vi "Initialize MeasurementLink Session.vi"(7 "remote connection options":T2, 8 "error in":errorcluster, 9 "initialize and close session behavior":T1, 10 "session initialization parameters":T3, 11 "session factory in":refnum<class "Session Factory.lvclass">) -> (0 "error out":errorcluster, 2 "session out":variant, 3 "session factory out":refnum<class "Session Factory.lvclass">)   [LabVIEW 2020, in "IVI Scope Instrument.lvlib" / "Session Factory.lvclass"]
doc: "Creates a new session using the provided <b>session initialization parameters</b>. If the session represents a remote session, <b>initialize and close session behavior</b> determines whether creating the local session creates a new session on the server or attaches to an existing session on the server."
uses:
  Session Factory.lvclass
  <vilib>/MeasurementLink/MeasurementLink Instrument/ISession Factory/Session Initialization Parameters.ctl
  <vilib>/MeasurementLink/MeasurementLink Instrument/ISession Factory/Remote Connection Options.ctl
  <vilib>/MeasurementLink/MeasurementLink Instrument/ISession Factory/Initialize and Close Session Behavior.ctl
  Session Factory.lvclass/Session Factory.ctl
  <vilib>/MeasurementLink/MeasurementLink Instrument/ISession Factory/ISession Factory.lvclass
  <vilib>/ivi/iviscope/_iviscope.llb/IviScope Initialize With Options.vi
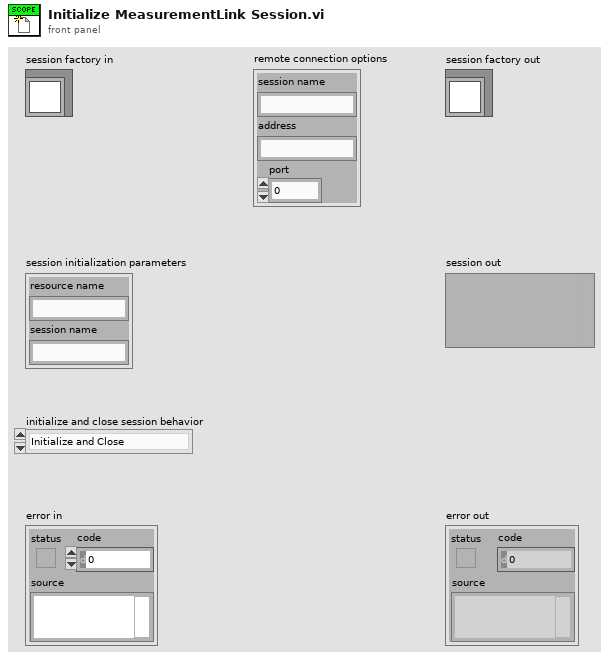
[diagram p1: front panel]
types:
  T1 = typedef "MeasurementLink Instrument.lvlib/ISession Factory.lvclass/Initialize and Close Session Behavior.ctl" = enum16{"Initialize and Close", "Attach and Detach", "Initialize and Detach", "Attach and Close"}
  T2 = typedef "MeasurementLink Instrument.lvlib/ISession Factory.lvclass/Remote Connection Options.ctl" = cluster{"session name":string, "address":string, "port":u32}
  T3 = typedef "MeasurementLink Instrument.lvlib/ISession Factory.lvclass/Session Initialization Parameters.ctl" = cluster{"resource name":string, "session name":string}
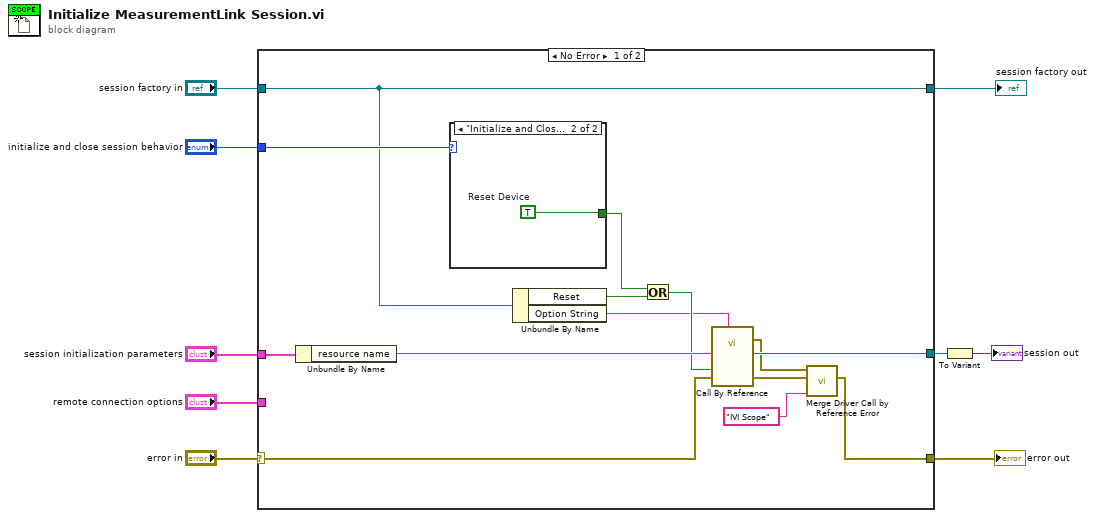
[diagram p0: block diagram]
diagram:
  n1 = case shown="No Error" "error in" {
    selector: "error in" -> [w16 w26]
    tunnel: [w13 w26] -> w8
    tunnel: [w11 w25] -> w7
    tunnel: "session factory in" -> [w11 w25]
    tunnel: "session initialization parameters" -> [w23 _]
    tunnel: [w21 _] -> w3
    tunnel: "initialize and close session behavior" -> [w20 _]
    tunnel: "remote connection options" -> [_ _]
    frame No Error {
      n2 = Unbundle By Name(w23) -> ("resource name"=w22:string)
      n3 = case shown="\"Initialize and Close\", \"Initialize and Detach\"" w20 {
        tunnel: [_ w24] -> w19
        frame Default {
        }
        frame "Initialize and Close", "Initialize and Detach" {
          w24 = TRUE  # Reset Device
        }
      }
      n4 = Unbundle By Name(w11) -> ("Reset"=w18:bool, "Option String"=w10:string)
      n5 = Or(x=w19, y=w18) -> (x .or. y?=w17:bool)
      n6 = call-by-ref "?"("option string (\"Simulate=0,RangeCheck=1,QueryInstrStatus=0,Cache=1\")"=w10, "error in (no error)"=w16, "reset device (True)"=w17, "logical name (\"SampleScope\")"=w22) -> (error out=w15:errorcluster, 0:"error out"=w14:errorcluster, "instrument handle out"=w21:refnum<k15>)  [unwired: 8 in, 1 out]
      n7 = call <vilib>:"Merge Driver Call by Reference Error.vi"("driver name"="IVI Scope", "called vi error"=w14, "call by ref error"=w15) -> ("error out"=w13:errorcluster)  [unwired: 8 in]
    }
    frame Error {
    }
  }
  "error out" <- w8
  "session factory out" <- w7
  n8 = To Variant(anything=w3) -> (Variant=→"session out":variant)
